vi "Get unique number.vi"() -> (0 "Globally unique number":i32)   [LabVIEW 2011, in "COSYLib.lvlib"]
doc: "Returns a different number each call.\n(This is a very simple Functional Global Variable)."
uses:
  COSYLib.lvlib
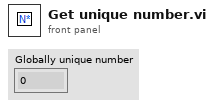
[diagram p1: front panel]
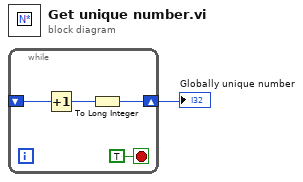
[diagram p0: block diagram]
diagram:
  n1 = while {
    shift-right: [w2] -> w1
    shift-left: _ -> [w3]
    stop <- TRUE stop-if-true
    n2 = Increment(x=w3) -> (x+1=w4:i32)
    n3 = To Long Integer(number=w4) -> (32bit integer=w2:i32)
  }
  "Globally unique number" <- w1
